vi "tm430_functions.vi"() -> ()   [LabVIEW 2011]
panel:
  out "Image":u16[][](graph)
  in  "Snap":bool
  in  "Parameter":u32(ring)=4212128 items=["SENSOR MODE"=4212128, "READOUT SPEED"=4211872, "READOUT DIRECTION"=4211904, "BIT PER CHANNEL"=4342976, "TRIGGER GLOBAL EXPOSURE"=2049680, "TRIGGER CONNECTOR"=1066432, "TRIGGER TIMES"=1066448, "SENSOR TEMPERATURE"=2115232, "EXPOSURE TIME"=2049184, "BINNING"=4215968, "TIMING READOUT TIME"=4223904, "IMAGE PIXEL TYPE"=4343296, "OUTPUT TRIGGER POLARITY[0]"=1852592, "OUTPUT TRIGGER POLARITY[1]"=1852848, "OUTPUT TRIGGER POLARITY[2]"=1853104, "OUTPUT TRIGGER DELAY[0]"=1852624, "OUTPUT TRIGGER DELAY[1]"=1852880, "OUTPUT TRIGGER DELAY[2]"=1853136, "OUTPUT TRIGGER PERIOD[0]"=1852640, "OUTPUT TRIGGER PERIOD[1]"=1852896, "OUTPUT TRIGGER PERIOD[2]"=1853152, "OUTPUT TRIGGER KIND[0]"=1852656, "OUTPUT TRIGGER KIND[1]"=1852912, "OUTPUT TRIGGER KIND[2]"=1853168]
  in  "Text Value":dbl(ring) items=["NEGATIVE"=1.0, "POSITIVE"=2.0]
  in  "Value":dbl(slide) min=1.0 max=2.0 scale=1.0..2.0
  out "error out":errorcluster
  in  "stop":bool
  # "This example shows a way you can access\nmany of the functions available to the camera and see how they affect the captured image."
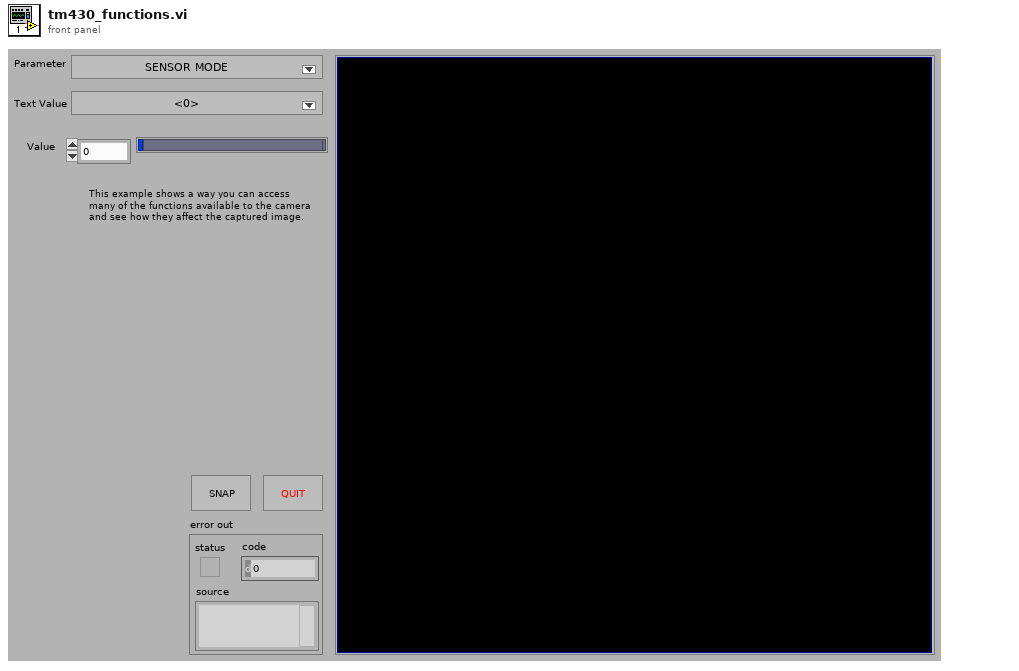
[diagram p1: front panel]
types:
  T1 = enum8{"Enabled", "Disabled", "Disabled and Grayed Out"}
  T2 = cluster{"Function Name":string, "Function ID":u32}[]
  T3 = cluster{"Function Name":string, "Function ID":u32}
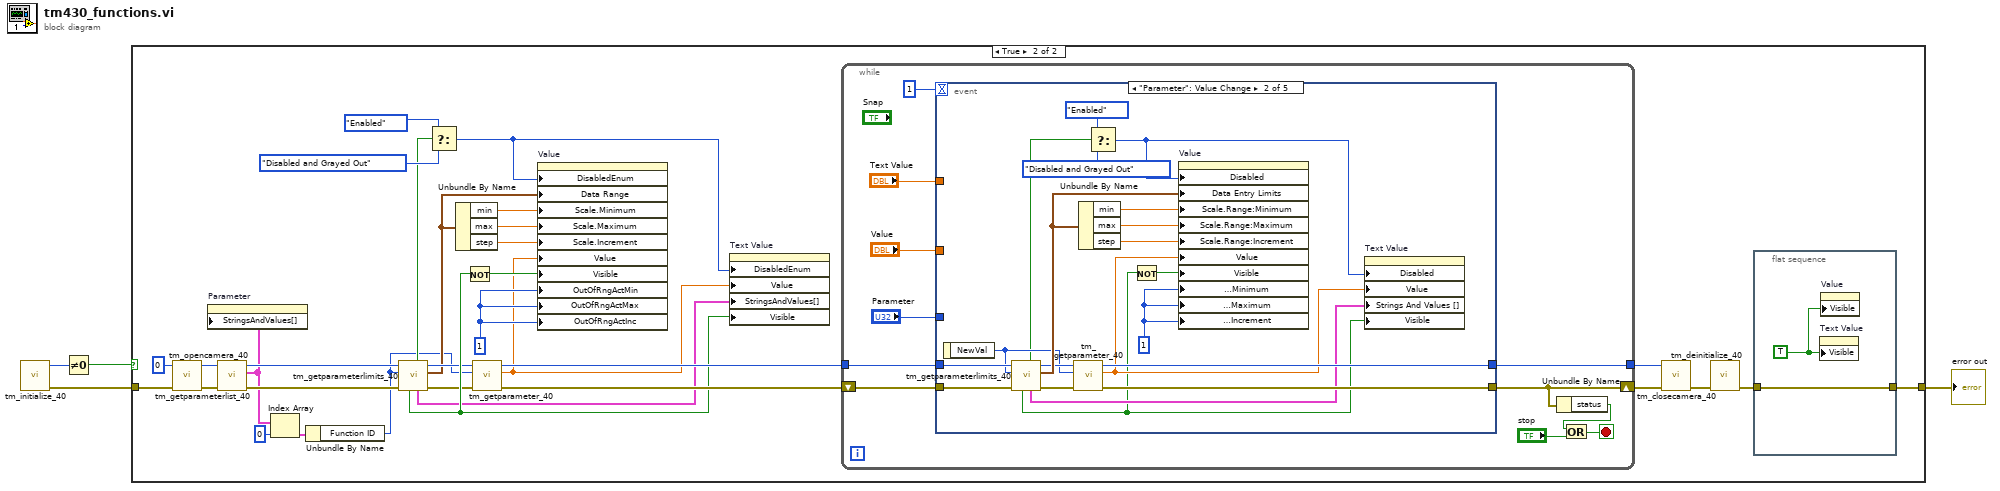
[diagram p0: block diagram]
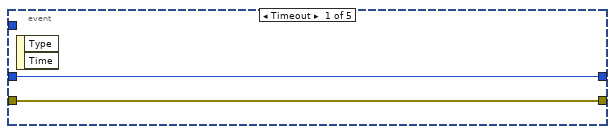
[diagram p3: hidden frame]
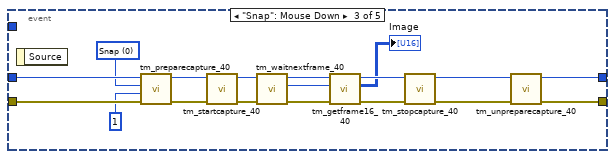
[diagram p4: hidden frame]
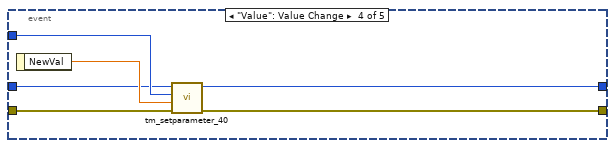
[diagram p5: hidden frame]
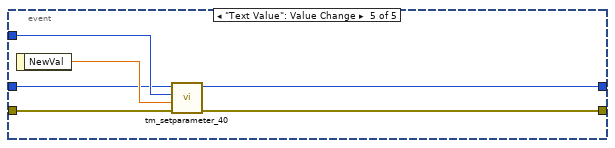
[diagram p6: hidden frame]
diagram:
  n1 = call <userlib>:"tm_initialize_40.vi"() -> ("error out"=w2:errorcluster, "Number Of Cameras"=w4:u32)  [unwired: 8 in, 2 out]
  n2 = Not Equal To 0?(x=w4) -> (x != 0?=w3:bool)
  n3 = case shown="True" w3 {
    tunnel: [w5 w32] -> w1
    tunnel: w2 -> [w5 w37]
    frame False {
    }
    frame True {
      w21 = u8 1 ("Out Of Range Action:Increment")
      n4 = call <userlib>:"tm_opencamera_40.vi"("error in (no error)"=w37, "Camera Index"=u32 0) -> ("error out"=w34:errorcluster, "Handle out"=w35:u32)  [unwired: 7 in, 1 out]
      n5 = call <userlib>:"tm_getparameterlist_40.vi"("error in (no error)"=w34, "Handle in"=w35) -> ("error out"=w16:errorcluster, "Function List"=w9:T2, "Handle out"=w17:u32)  [unwired: 7 in]
      n6 = property on="Parameter" class="Ring (strict)"("StringsAndValues[]"=w9) -> ()  [unwired: 2 in, 2 out]
      n7 = Index Array(array=w9, index=0) -> (element=w7:T3)
      n8 = Unbundle By Name(w7) -> ("Function ID"=w6:u32)
      n9 = call <userlib>:"tm_getparameterlimits_40.vi"("error in (no error)"=w16, "Parameter"=w6, "Handle in"=w17) -> ("error out"=w10:errorcluster, "Range"=w11:cluster{"min":dbl, "max":dbl, "step":dbl}, "Handle out"=w12:u32, "Value Names"=w14:cluster{"Name":string, "Value":dbl}[], "Writable"=w13:bool, "Text Values"=w15:bool)  [unwired: 2 in, 1 out]
      n10 = Select(t=T1."Enabled" ("Disabled"), s=w13, f=T1."Disabled and Grayed Out" ("Disabled")) -> (s? t:f=w26:T1)
      n11 = Unbundle By Name(w11) -> ("min"=w25:dbl, "max"=w24:dbl, "step"=w23:dbl)
      n12 = Not(x=w15) -> (.not. x?=w22:bool)
      n13 = call <userlib>:"tm_getparameter_40.vi"("error in (no error)"=w10, "Parameter"=w6, "Handle in"=w12) -> ("error out"=w18:errorcluster, "Value out"=w19:dbl, "Handle out"=w20:u32)  [unwired: 6 in]
      n14 = property on="Value" class="Slide (strict)"("DisabledEnum"=w26, "Data Range"=w11, "Scale.Minimum"=w25, "Scale.Maximum"=w24, "Scale.Increment"=w23, "Value"=w19, "Visible"=w22, "OutOfRngActMin"=w21, "OutOfRngActMax"=w21, "OutOfRngActInc"=w21) -> ()  [unwired: 2 in, 2 out]
      n15 = property on="Text Value" class="Ring (strict)"("DisabledEnum"=w26, "Value"=w19, "StringsAndValues[]"=w14, "Visible"=w15) -> ()  [unwired: 2 in, 2 out]
      n16 = while {
        tunnel: w20 -> [w46]
        tunnel: [w44] -> w30
        shift-right: [w43] -> w31
        shift-left: w18 -> [w47]
        stop <- w48 stop-if-true
        n17 = event shown="[1] \"Parameter\": Value Change" {
          selector: _ -> [_ _ _ _ _]
          dyn-events: _ -> [_ _ _ _ _]
          timeout: 1 -> [_ _ _ _ _]
          tunnel: w47 -> [w52 w60 w89 w96 w102]
          tunnel: w46 -> [w51 w61 w90 w93 w98]
          tunnel: [w51 w64 w80 w92 w97] -> w44
          tunnel: [w52 w62 w79 w91 w101] -> w43
          tunnel: "Parameter" -> [_ _ _ w94 w99]
          tunnel: "Value" -> [_ _ _ _ _]
          tunnel: "Text Value" -> [_ _ _ _ _]
          event Timeout {
            n18 = event-data() -> ()  [unwired: 1 in, 2 out]
          }
          event "Parameter": Value Change {
            w68 = u8 1 ("Out Of Range Action:Increment")
            n19 = event-data() -> ("NewVal"=w55:u32)  [unwired: 1 in]
            n20 = call <userlib>:"tm_getparameterlimits_40.vi"("error in (no error)"=w60, "Parameter"=w55, "Handle in"=w61) -> ("error out"=w58:errorcluster, "Range"=w57:cluster{"min":dbl, "max":dbl, "step":dbl}, "Handle out"=w56:u32, "Value Names"=w59:cluster{"Name":string, "Value":dbl}[], "Writable"=w53:bool, "Text Values"=w54:bool)  [unwired: 2 in, 1 out]
            n21 = call <userlib>:"tm_getparameter_40.vi"("error in (no error)"=w58, "Parameter"=w55, "Handle in"=w56) -> ("error out"=w62:errorcluster, "Value out"=w63:dbl, "Handle out"=w64:u32)  [unwired: 6 in]
            n22 = Unbundle By Name(w57) -> ("min"=w72:dbl, "max"=w71:dbl, "step"=w70:dbl)
            n23 = Select(t=T1."Enabled" ("Disabled"), s=w53, f=T1."Disabled and Grayed Out" ("Disabled")) -> (s? t:f=w67:T1)
            n24 = Not(x=w54) -> (.not. x?=w69:bool)
            n25 = property on="Value" class="Slide (strict)"("Disabled"=w67, "Data Entry Limits"=w57, "Scale.Range:Minimum"=w72, "Scale.Range:Maximum"=w71, "Scale.Range:Increment"=w70, "Value"=w63, "Visible"=w69, "Response to Value Outside Limits:Minimum"=w68, "Response to Value Outside Limits:Maximum"=w68, "Response to Value Outside Limits:Increment"=w68) -> ()  [unwired: 2 in, 2 out]
            n26 = property on="Text Value" class="Ring (strict)"("Disabled"=w67, "Value"=w63, "Strings And Values []"=w59, "Visible"=w54) -> ()  [unwired: 2 in, 2 out]
          }
          event "Snap": Mouse Down {
            w88 = 0 items=["Snap", "Sequence"] ("Capture mode")
            n27 = event-data() -> ()  [unwired: 1 in, 1 out]
            n28 = call <userlib>:"tm_preparecapture_40.vi"("error in (no error)"=w89, "Frames"=1, "Capture mode"=w88, "Handle in"=w90) -> ("error out"=w86:errorcluster, "Handle out"=w85:u32)  [unwired: 4 in, 2 out]
            n29 = call <userlib>:"tm_startcapture_40.vi"("error in (no error)"=w86, "Handle in"=w85) -> ("error out"=w77:errorcluster, "Handle out"=w78:u32)  [unwired: 8 in]
            n30 = call <userlib>:"tm_waitnextframe_40.vi"("error in (no error)"=w77, "Handle in"=w78) -> ("error out"=w75:errorcluster, "Frame Index"=w73:i32, "Handle out"=w76:u32)  [unwired: 6 in, 1 out]
            n31 = call <userlib>:"tm_getframe16_40.vi"("error in (no error)"=w75, "Frame Index"=w73, "Handle in"=w76) -> ("error out"=w83:errorcluster, "Data"=→"Image":u16[][], "Handle out"=w84:u32)  [unwired: 5 in, 1 out]
            n32 = call <userlib>:"tm_stopcapture_40.vi"("error in (no error)"=w83, "Handle in"=w84) -> ("error out"=w82:errorcluster, "Handle out"=w81:u32)  [unwired: 8 in]
            n33 = call <userlib>:"tm_unpreparecapture_40.vi"("error in (no error)"=w82, "Handle in"=w81) -> ("error out"=w79:errorcluster, "Handle out"=w80:u32)  [unwired: 8 in]
          }
          event "Value": Value Change {
            n34 = event-data() -> ("NewVal"=w95:dbl)  [unwired: 1 in]
            n35 = call <userlib>:"tm_setparameter_40.vi"("error in (no error)"=w96, "Value in"=w95, "Parameter"=w94, "Handle in"=w93) -> ("error out"=w91:errorcluster, "Handle out"=w92:u32)  [unwired: 6 in]
          }
          event "Text Value": Value Change {
            n36 = event-data() -> ("NewVal"=w100:dbl)  [unwired: 1 in]
            n37 = call <userlib>:"tm_setparameter_40.vi"("error in (no error)"=w102, "Value in"=w100, "Parameter"=w99, "Handle in"=w98) -> ("error out"=w101:errorcluster, "Handle out"=w97:u32)  [unwired: 6 in]
          }
        }
        n38 = Unbundle By Name(w43) -> ("status"=w49:bool)
        n39 = Or(x=w49, y="stop") -> (x .or. y?=w48:bool)
      }
      n40 = call <userlib>:"tm_closecamera_40.vi"("error in (no error)"=w31, "Handle in"=w30) -> ("error out"=w36:errorcluster)  [unwired: 9 in]
      n41 = call <userlib>:"tm_deinitialize_40.vi"("error in (no error)"=w36) -> ("error out"=w33:errorcluster)  [unwired: 10 in]
      n42 = flat-sequence {
        tunnel: w33 -> [w39]
        tunnel: [w39] -> w32
        frame #0 {
          w38 = TRUE
          n43 = property on="Text Value" class="Ring (strict)"("Visible"=w38) -> ()  [unwired: 2 in, 2 out]
          n44 = property on="Value" class="Slide (strict)"("Visible"=w38) -> ()  [unwired: 2 in, 2 out]
        }
      }
    }
  }
  "error out" <- w1
